vi "1553B-RECV-START.vi"(8 "错误输入（无错误）":errorcluster, 9 "Zhufen/Beifen":string(combo), 10 "Zhufei/Beifen":bool, 11 "字节流文件输入":refnum<file>) -> (0 "错误输出":errorcluster)   [LabVIEW 2012]
uses:
  <vilib>/GPower/VIRegister/Library/Convert/ToU8.vi
  <vilib>/GPower/VIRegister/Library/Convert/ToStr.vi
  <vilib>/GPower/VIRegister/Library/Convert/ToU32.vi
  <vilib>/GPower/VIRegister/Library/SubVIs/FindRegisterData.vi
  <vilib>/GPower/VIRegister/Library/SubVIs/ReadSub.vi
  <vilib>/GPower/VIRegister/Library/SubVIs/WriteSub.vi
  <vilib>/GPower/VIRegister/Library/QManager/GetRegisterData.vi
  <vilib>/GPower/Error/Library/SetError.vi
  <vilib>/GPower/Error/Library/FilterCodes.vi
  <vilib>/GPower/Error/Library/Filter/FilterMulti.vi
  <vilib>/GPower/VIRegister/Library/QManager/QManagerAction.vi
  <vilib>/GPower/Error/Library/ErrorType.vi
  <vilib>/GPower/Error/Library/SplitAppended.vi
  <vilib>/GPower/Error/Library/SubVIs/ExplanationToError.vi
  <vilib>/GPower/VIRegister/Library/QManager/GetQName.vi
  <vilib>/GPower/VIRegister/Library/QManager/StartQManager.vi
  <vilib>/Utility/error.llb/Trim Whitespace.vi
  <vilib>/dlg_ctls.llb/Space Constant.vi
  <vilib>/Utility/error.llb/Error Code Database.vi
  <vilib>/GPower/Error/Library/SubVIs/SetStatus.vi
  <vilib>/GPower/Error/Library/AppendErrors.vi
  <vilib>/GPower/Error/Library/Append/AppendSingle.vi
  <vilib>/GPower/VIRegister/VIRegister.lvlib
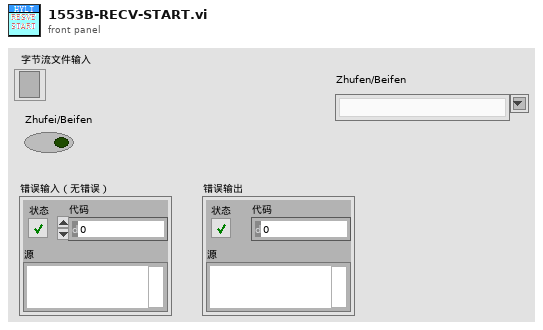
[diagram p1: front panel]
types:
  T1 = cluster{"G1陀螺脉冲数":i32, "G2陀螺脉冲数":i32, "G3陀螺脉冲数":i32, "A1加速度计脉冲数":i16, "A2加速度计脉冲数":i16, "A3加速度计脉冲数":i16, "G1陀螺自检状态":u8, "G1陀螺光路温度":i8, "G2陀螺自检状态":u8, "G2陀螺光路温度":i8, "G3陀螺自检状态":u8, "G3陀螺光路温度":i8, "A1自检状态":u8, "A1幅值":u8, "A2自检状态":u8, "A2幅值":u8, "A3自检状态":u8, "A3幅值":u8, "IF1电路温度":i8, "IF2电路温度":i8, "IF3电路温度":i8, "温控自检字":u8, "加计温度1":i16, "加计温度2":i16, "LTU状态":u8, "帧计数":u8}
  T2 = cluster{"G1陀螺脉冲数":i32, "G2陀螺脉冲数":i32, "G3陀螺脉冲数":i32, "A1加速度计脉冲数":i32, "A2加速度计脉冲数":i32, "A3加速度计脉冲数":i32, "G1陀螺光路温度":u8, "G2陀螺光路温度":u8, "G3陀螺光路温度":u8, "加计温度1":u8, "加计温度2":u8, "帧计数":u8, "自检状态_v4":u8, "脉冲累计时间的整数值_v4":u16}
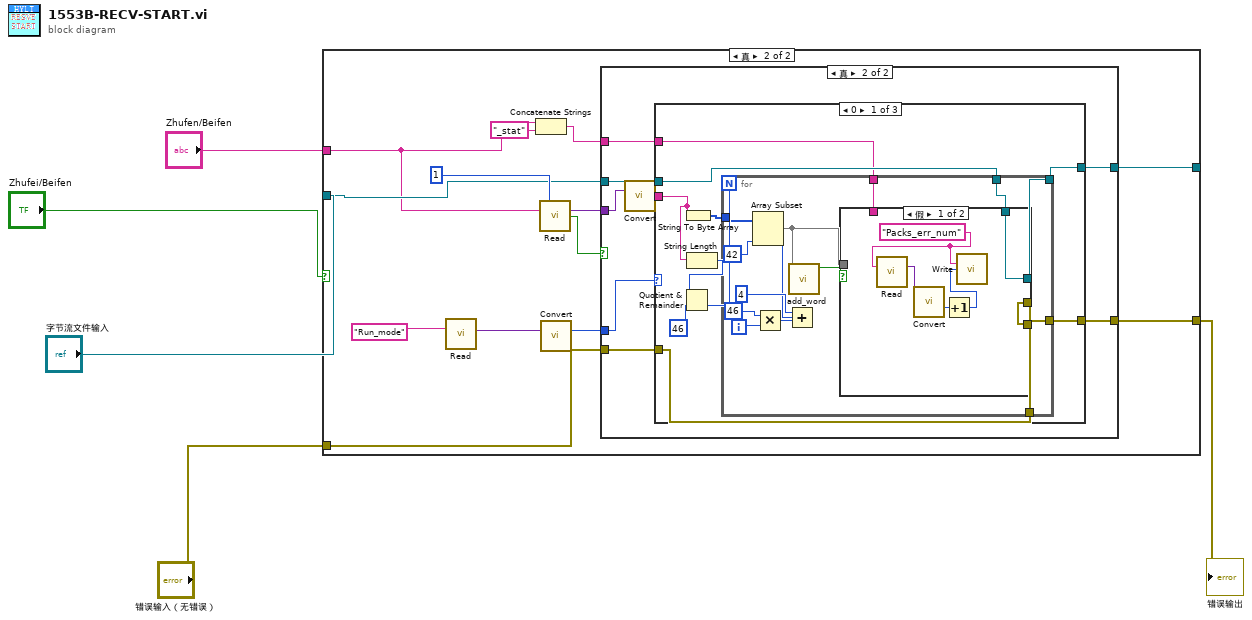
[diagram p0: block diagram]
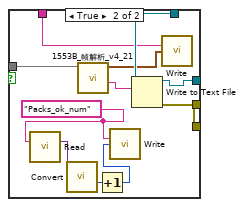
[diagram p4: hidden frame]
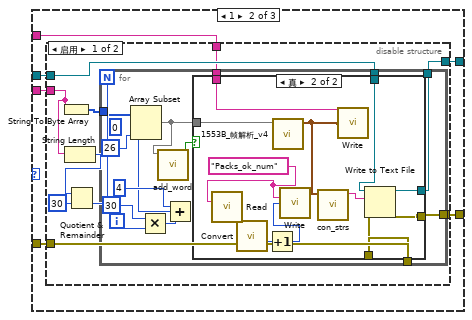
[diagram p5: hidden frame]
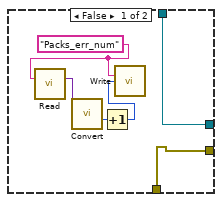
[diagram p6: hidden frame]
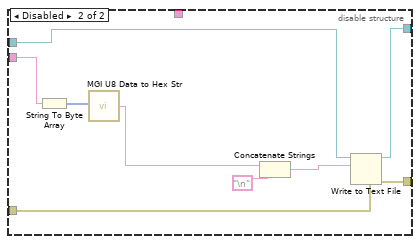
[diagram p7: hidden frame]
diagram:
  n1 = case shown="真" "Zhufei/Beifen" {
    tunnel: "字节流文件输入" -> [w6 w13]
    tunnel: "错误输入（无错误）" -> [w7 w12]
    tunnel: [w7 w11] -> w5
    tunnel: [w6 w15] -> _
    tunnel: "Zhufen/Beifen" -> [_ w10]
    frame False {
    }
    frame True {
      n2 = call <vilib>:"Read.vi"("Register name"="Run_mode") -> ("Register value"=w16:variant)  [unwired: 11 in, 3 out]
      n3 = Concatenate Strings(w10, "_stat" ("字符串")) -> (w8:string)
      n4 = call <vilib>:"Read.vi"("Timeout"=1, "Register name"=w10) -> ("Register value"=w19:variant, "Register value read?"=w20:bool)  [unwired: 10 in, 2 out]
      n5 = call-poly <vilib>:"Convert.vi"("Register value in"=w16) -> ("Register value out"=w14:u8)  [unwired: 13 in, 1 out]
      n6 = case shown="真" w20 {
        tunnel: w19 -> [_ w30]
        tunnel: w13 -> [w21 w28]
        tunnel: w14 -> [_ w27]
        tunnel: w12 -> [w22 w26]
        tunnel: [w22 w25] -> w11
        tunnel: [w21 w24] -> w15
        tunnel: w8 -> [_ w23]
        frame False {
        }
        frame True {
          n7 = call-poly <vilib>:"Convert.vi"("Register value in"=w30) -> ("Register value out"=w29:string)  [unwired: 13 in, 1 out]
          n8 = case shown="0" w27 {
            tunnel: w29 -> [w35 w74 _]
            tunnel: w28 -> [w39 w78 w131]
            tunnel: w26 -> [w38 w77 w130]
            tunnel: [w37 w76 w130] -> w25
            tunnel: [w36 w75 w131] -> w24
            tunnel: w23 -> [w31 w73 _]
            frame 0 {
              n9 = String To Byte Array(string=w35) -> (unsigned byte array=w40:u8[])
              n10 = String Length(string=w35) -> (length=w34:i32)
              n11 = Quotient & Remainder(x=w34, y=46) -> (floor(x/y)=w32:i32)  [unwired: 1 out]
              n12 = for {
                N: w32 -> [_]
                tunnel: w40 -> [w44]
                tunnel: w39 -> [w53]
                tunnel: w38 -> [w52]
                tunnel: [w51] -> w37
                tunnel: [w50] -> w36
                tunnel: w31 -> [w41]
                i -> [w49]
                n13 = Multiply(x=46, y=w49) -> (x*y=w47:i32)
                n14 = Add(x=4 ("索引"), y=w47) -> (x+y=w45:i32)
                n15 = Array Subset(array=w44, index=w45, length=42 ("长度")) -> (w43:u8[])
                n16 = call "add_word.vi"("子数组"=w43) -> ("校验通过"=w42:bool)  [unwired: 10 in]
                n17 = case shown="假" w42 {
                  tunnel: w53 -> [w60 w72]
                  tunnel: w43 -> [_ w71]
                  tunnel: w52 -> [w59 w68]
                  tunnel: [w59 w67] -> w51
                  tunnel: [w60 w66] -> w50
                  tunnel: w41 -> [_ w61]
                  frame False {
                    w58 = "Packs_err_num" ("Register name")
                    n18 = call <vilib>:"Read.vi"("Register name"=w58) -> ("Register value"=w57:variant)  [unwired: 11 in, 3 out]
                    n19 = call-poly <vilib>:"Convert.vi"("Register value in"=w57) -> ("Register value out"=w56:u32)  [unwired: 13 in, 1 out]
                    n20 = Increment(x=w56) -> (x+1=w55:u32)
                    n21 = call <vilib>:"Write.vi"("Register name"=w58, "Register value"=w55) -> ()  [unwired: 11 in, 3 out]
                  }
                  frame True {
                    w65 = "Packs_ok_num" ("Register name")
                    n22 = call <vilib>:"Read.vi"("Register name"=w65) -> ("Register value"=w64:variant)  [unwired: 11 in, 3 out]
                    n23 = call-poly <vilib>:"Convert.vi"("Register value in"=w64) -> ("Register value out"=w63:u32)  [unwired: 13 in, 1 out]
                    n24 = call "1553B_帧解析_v4_21.vi"("数组"=w71) -> ("连接的字符串"=w70:string, "输出簇"=w69:T1)  [unwired: 9 in]
                    n25 = Increment(x=w63) -> (x+1=w62:u32)
                    n26 = call <vilib>:"Write.vi"("Register name"=w65, "Register value"=w62) -> ()  [unwired: 11 in, 3 out]
                    n27 = Write to Text File(file (use dialog)=w72, text=w70, error in=w68) -> (refnum out=w66:refnum<file>, error out=w67:errorcluster)  [unwired: 1 in, 1 out]
                    n28 = call <vilib>:"Write.vi"("Register name"=w61, "Register value"=w69) -> ()  [unwired: 11 in, 3 out]
                  }
                }
              }
            }
            frame 1 {
              n29 = disable-structure shown="启用" {
                disable-tunnel: w78 -> [w87 w129]
                disable-tunnel: w77 -> [w86 w128]
                disable-tunnel: [w85 w127] -> w76
                disable-tunnel: [w84 w126] -> w75
                disable-tunnel: w74 -> [w83 w125]
                disable-tunnel: w73 -> [w79 _]
                frame Enabled {
                  n30 = String To Byte Array(string=w83) -> (unsigned byte array=w88:u8[])
                  n31 = String Length(string=w83) -> (length=w82:i32)
                  n32 = Quotient & Remainder(x=w82, y=30) -> (floor(x/y)=w80:i32)  [unwired: 1 out]
                  n33 = for {
                    N: w80 -> [_]
                    tunnel: w88 -> [w93]
                    tunnel: w87 -> [w101]
                    tunnel: w86 -> [w91]
                    tunnel: [w100] -> w85
                    tunnel: [w99] -> w84
                    tunnel: w79 -> [w89]
                    i -> [w98]
                    (unwired) 0 ("索引")
                    n34 = Multiply(x=30, y=w98) -> (x*y=w96:i32)
                    n35 = Add(x=4 ("索引"), y=w96) -> (x+y=w94:i32)
                    n36 = Array Subset(array=w93, index=w94, length=26 ("长度")) -> (w92:u8[])
                    n37 = call "add_word.vi"("子数组"=w92) -> ("校验通过"=w90:bool)  [unwired: 10 in]
                    n38 = case shown="真" w90 {
                      tunnel: w101 -> [w108 w120]
                      tunnel: [w107 w119] -> w100
                      tunnel: [w108 w118] -> w99
                      tunnel: w92 -> [_ w115]
                      tunnel: w91 -> [w107 w114]
                      tunnel: w89 -> [_ w109]
                      frame False {
                        w106 = "Packs_err_num" ("Register name")
                        n39 = call <vilib>:"Read.vi"("Register name"=w106) -> ("Register value"=w105:variant)  [unwired: 11 in, 3 out]
                        n40 = call-poly <vilib>:"Convert.vi"("Register value in"=w105) -> ("Register value out"=w104:u32)  [unwired: 13 in, 1 out]
                        n41 = Increment(x=w104) -> (x+1=w103:u32)
                        n42 = call <vilib>:"Write.vi"("Register name"=w106, "Register value"=w103) -> ()  [unwired: 11 in, 3 out]
                      }
                      frame True {
                        w110 = "Packs_ok_num" ("Register name")
                        n43 = call <vilib>:"Read.vi"("Register name"=w110) -> ("Register value"=w113:variant)  [unwired: 11 in, 3 out]
                        n44 = call-poly <vilib>:"Convert.vi"("Register value in"=w113) -> ("Register value out"=w112:u32)  [unwired: 13 in, 1 out]
                        n45 = Increment(x=w112) -> (x+1=w111:u32)
                        n46 = call "1553B_帧解析_v4.vi"("数组"=w115) -> ("输出簇"=w117:T2)  [unwired: 10 in]
                        n47 = call <vilib>:"Write.vi"("Register name"=w110, "Register value"=w111) -> ()  [unwired: 11 in, 3 out]
                        n48 = call "con_strs.vi"("输出簇"=w117) -> ("连接的字符串"=w116:string)  [unwired: 10 in]
                        n49 = call <vilib>:"Write.vi"("Register name"=w109, "Register value"=w117) -> ()  [unwired: 11 in, 3 out]
                        n50 = Write to Text File(file (use dialog)=w120, text=w116, error in=w114) -> (refnum out=w118:refnum<file>, error out=w119:errorcluster)  [unwired: 1 in, 1 out]
                      }
                    }
                  }
                }
                frame Disabled {
                  n51 = String To Byte Array(string=w125) -> (unsigned byte array=w124:u8[])
                  n52 = call <userlib>:"MGI U8 Data to Hex Str.vi"("u8 Data[]"=w124) -> ("HEX String (0-9,A-F)"=w123:string)
                  n53 = Concatenate Strings(w123, "\n") -> (w122:string)
                  n54 = Write to Text File(file (use dialog)=w129, text=w122, error in=w128) -> (refnum out=w126:refnum<file>, error out=w127:errorcluster)  [unwired: 1 in, 1 out]
                }
              }
            }
            frame 2, Default {
            }
          }
        }
      }
    }
  }
  "错误输出" <- w5
